vi "GetClass.vi"() -> (3 "Classes":string[](array[string]))   [LabVIEW 2020]
uses:
  Classes/Osciloscope/Osciloscope.lvclass
  Classes/TektronicsTDS/TektroniksTDS.lvclass
  C:/Users/HP/Documents/7mo/Instrumentacion/Parcial2/Osciloscope/Osciloscopio_DuranMu-oz/OsciloscopioProject/Classes/Osciloscope/Osciloscope.lvclass
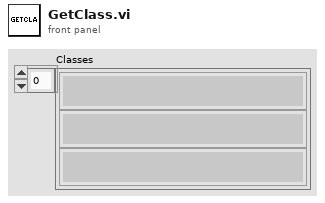
[diagram p1: front panel]
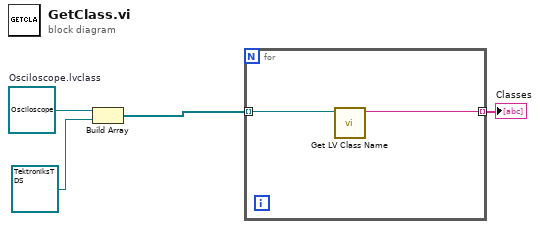
[diagram p0: block diagram]
diagram:
  w2 = refnum<class "Osciloscope.lvclass"> refnum  # Osciloscope.lvclass
  n1 = Build Array(w2, refnum<class "TektroniksTDS.lvclass"> refnum ("TektroniksTDS.lvclass")) -> (w4:refnum<class "Osciloscope.lvclass">[])
  n2 = for {
    tunnel: w4 -> [w6] mode=indexing
    tunnel: [w5] -> w3 mode=indexing
    n3 = call <vilib>:"Get LV Class Name.vi"("object"=w6) -> ("class name"=w5:string)  [unwired: 9 in, 1 out]
  }
  "Classes" <- w3
